vi "LUT.grey-progress.vi"() -> (0 "grey-progress":cluster{u8, u8, u8}[](array[cluster]))   [LabVIEW 2013]
panel:
  in  "gamma":dbl=0.5 format="%.2f"
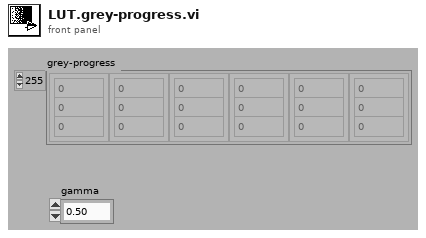
[diagram p1: front panel]
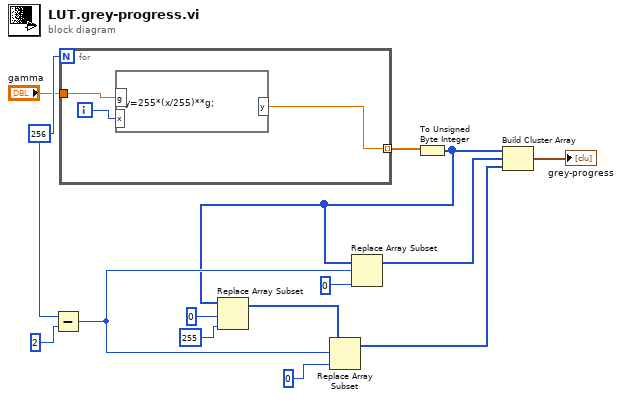
[diagram p0: block diagram]
diagram:
  w14 = 256
  n1 = Subtract(x=w14, y=u8 2) -> (x-y=w10:i32)
  n2 = for {
    N: w14 -> [_]
    tunnel: [w17] -> w1 mode=indexing
    tunnel: "gamma" -> [w15]
    i -> [w16]
    n3 = formula code="y=255*(x/255)**g;"("x"=w16, "g"=w15) -> ("y"=w17:dbl)
  }
  n4 = To Unsigned Byte Integer(number=w1) -> (unsigned 8bit integer=w2:u8[])
  n5 = Replace Array Subset(array=w2, new element=255, index=0) -> (w8:u8[])
  n6 = Replace Array Subset(array=w8, new element=0, index=w10) -> (w7:u8[])
  n7 = Replace Array Subset(array=w2, new element=0, index=w10) -> (w6:u8[])
  n8 = Build Cluster Array(w2, w6, w7) -> (→"grey-progress":cluster{"y":u8, "y":u8, "y":u8}[])
